vi "Untitled 1.vi"() -> ()   [LabVIEW 2019]
uses:
  lib/Keithley 622x/Keithley 622x.lvlib
panel:
  out "Offset Past Token":i32
  out "Measurement 2":dbl
  out "Measurement Metadata 2":T1
  out "2182-A Reponse String":string
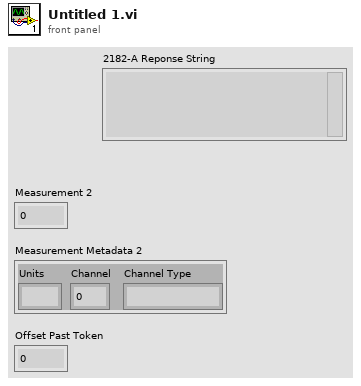
[diagram p1: front panel]
types:
  T1 = cluster{"Units":string, "Channel":i32, "Channel Type":string}
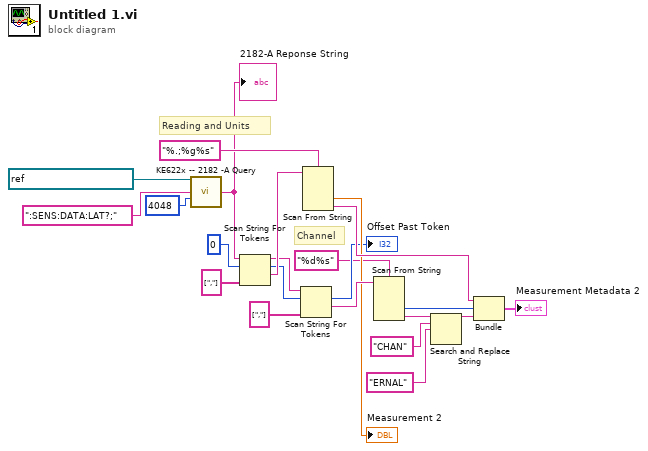
[diagram p0: block diagram]
diagram:
  # "Channel"
  # "Reading and Units"
  n1 = call "KE622x -- 2182 -A Query.vi"("622x Resource In"=refnum<visa-resource-name> "GPIB1::10::INSTR", "2182-A Write String"=":SENS:DATA:LAT?;" ("write buffer"), "Max Num Bytes To Read (256)"=u32 4048) -> ("2182-A Reponse String"=w2:string)  [unwired: 10 in, 2 out]
  "2182-A Reponse String" <- w2
  n2 = Scan String For Tokens(6:string[] [","] ("delimiters (\\s,\\t,\\r,\\n)"), 8:0 ("offset"), 9:w2) -> (1:w18:string, 2:w15:i32, 3:w17:string)  [unwired: 3 in, 1 out]
  n3 = Scan String For Tokens(6:string[] [","] ("delimiters (\\s,\\t,\\r,\\n)"), 8:w15, 9:w17) -> (1:w13:string, 2:→"Offset Past Token":i32)  [unwired: 3 in, 2 out]
  n4 = Scan From String(format string="%.;%g%s", input string=w18) -> (output 1=→"Measurement 2":dbl, output 2=w14:string)  [unwired: 4 in, 3 out]
  n5 = Scan From String(format string="%d%s", input string=w13) -> (output 1=w12:i32, output 2=w11:string)  [unwired: 4 in, 3 out]
  n6 = Search and Replace String(input string=w11, search string="CHAN", replace string="ERNAL" ("replace string (\"\")")) -> (result string=w8:string)  [unwired: 5 in, 3 out]
  n7 = Bundle(w14, w12, "result string"=w8) -> (→"Measurement Metadata 2":cluster{string, i32, "result string":string})  [unwired: 1 in]
